vi "ProcessName.vi"() -> (1 "process name":string="EmsaDataFlowManager")   [LabVIEW 2017, in "EmsaDataFlowManager.lvlib"]
uses:
  <vilib>/addons/InsightCM/Devices/Shared/Emsa/EmsaDataFlowManager/EmsaDataFlowManager.lvlib
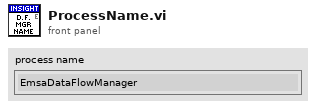
[diagram p1: front panel]
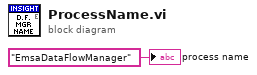
[diagram p0: block diagram]
diagram:
  "process name" <- "EmsaDataFlowManager" ("ProcessName")
